vi "makeDecisions.vi"(8 "error in (no error)":errorcluster, 10 "model":refnum<class "Model.lvclass">, 11 "EnabledState in":refnum<class "EnabledState.lvclass">) -> (0 "error out":errorcluster, 2 "model 2":refnum<class "Model.lvclass">, 3 "EnabledState out":refnum<class "EnabledState.lvclass">)   [LabVIEW 2013, in "EnabledState.lvclass"]
uses:
  EnabledState.lvclass
  Model/Model/Model.lvclass
  Typedefs/StateSelector.ctl
  Typedefs/FAMTTypedefs.lvlib
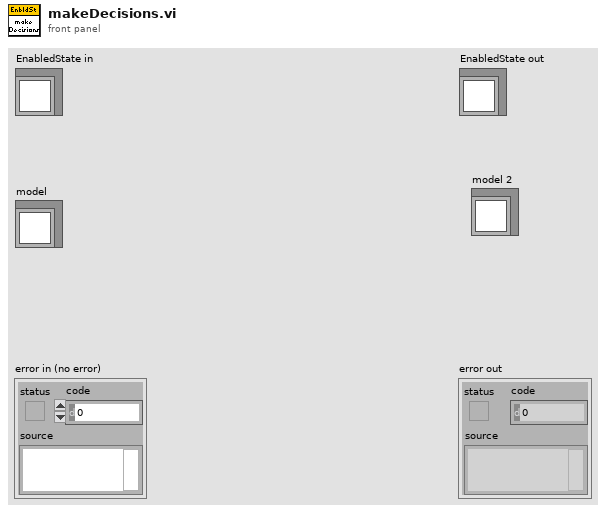
[diagram p1: front panel]
types:
  T1 = typedef "FAMTTypedefs.lvlib/StateSelector.ctl" = enum16{"EndingCycleState", "FaultState", "InteractiveSetpointState", "OffState", "StandbyState", "StoppedState"}
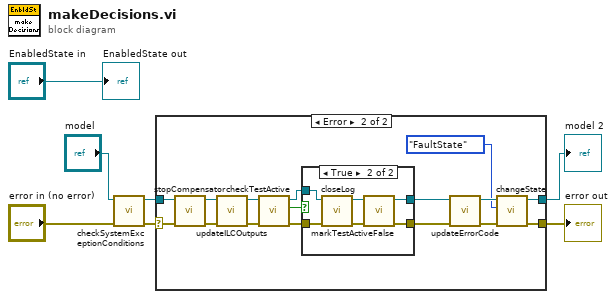
[diagram p0: block diagram]
diagram:
  n1 = call "checkSystemExceptionConditions.vi"("error in (no error)"="error in (no error)", "Model in"="model") -> ("error out"=w4:errorcluster, "Model out"=w3:refnum<class "Model.lvclass">)  [unwired: 8 in]
  n2 = case shown="Error" w4 {
    selector: w4 -> [w9 w19]
    tunnel: [w9 w23] -> w7
    tunnel: w3 -> [w8 w20]
    tunnel: [w8 w22] -> w5
    frame No Error {
    }
    frame Error {
      n3 = call "stopCompensator.vi"("error in (no error)"=w19, "Model in"=w20) -> ("error out"=w12:errorcluster, "Model out"=w13:refnum<class "Model.lvclass">)  [unwired: 8 in]
      n4 = call "updateILCOutputs.vi"("error in (no error)"=w12, "Model in"=w13) -> ("error out"=w10:errorcluster, "Model out"=w11:refnum<class "Model.lvclass">)  [unwired: 8 in]
      n5 = call "checkTestActive.vi"("error in (no error)"=w10, "Model in"=w11) -> ("error out"=w16:errorcluster, "testActiveIsTrue"=w18:bool, "Model out"=w17:refnum<class "Model.lvclass">)  [unwired: 7 in]
      n6 = case shown="True" w18 {
        tunnel: [w27 w30] -> w14
        tunnel: [w26 w28] -> w15
        tunnel: w17 -> [w27 w33]
        tunnel: w16 -> [w26 w32]
        frame False {
        }
        frame True {
          n7 = call "closeLog.vi"("error in (no error)"=w32, "Model in"=w33) -> ("error out"=w29:errorcluster, "Model out"=w31:refnum<class "Model.lvclass">)  [unwired: 8 in]
          n8 = call "markTestActiveFalse.vi"("error in (no error)"=w29, "Model in"=w31) -> ("error out"=w28:errorcluster, "Model out"=w30:refnum<class "Model.lvclass">)  [unwired: 8 in]
        }
      }
      n9 = call "updateErrorCode.vi"("error in (no error)"=w15, "Model in"=w14) -> ("error out"=w24:errorcluster, "Model out"=w25:refnum<class "Model.lvclass">)  [unwired: 8 in]
      n10 = call "changeState.vi"("error in (no error)"=w24, "State:"=StateSelector."FaultState", "Model in"=w25) -> ("error out"=w23:errorcluster, "Model out"=w22:refnum<class "Model.lvclass">)  [unwired: 7 in]
    }
  }
  "error out" <- w7
  "model 2" <- w5
  "EnabledState out" <- "EnabledState in"
